vi "Write Test Stand.vi"(8 "error in (no error)":errorcluster, 10 "Generic Test Stand.lvclass":refnum<class "Generic Test Stand.lvclass">, 11 "Run DAC Front Panel in":refnum<class "Run DAC Front Panel.lvclass">) -> (0 "error out":errorcluster, 3 "Run DAC Front Panel out":refnum<class "Run DAC Front Panel.lvclass">)   [LabVIEW 2019, in "DAC Process.lvlib" / "Run DAC Front Panel.lvclass"]
uses:
  Run DAC Front Panel.lvclass
  Generic Test Stand/Generic Test Stand.lvclass
  Run DAC Front Panel.lvclass/Run DAC Front Panel.ctl
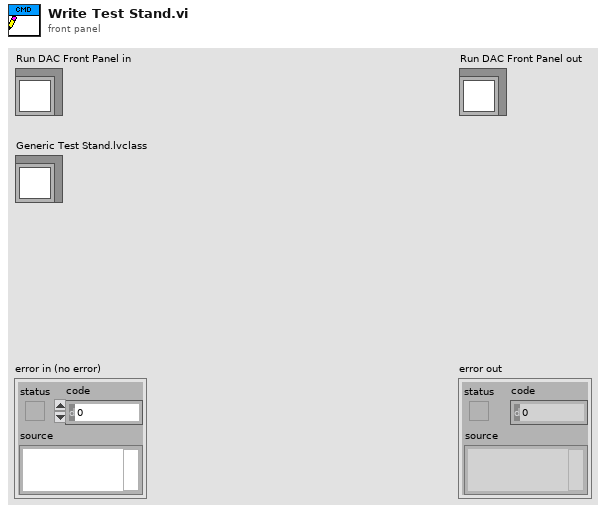
[diagram p1: front panel]
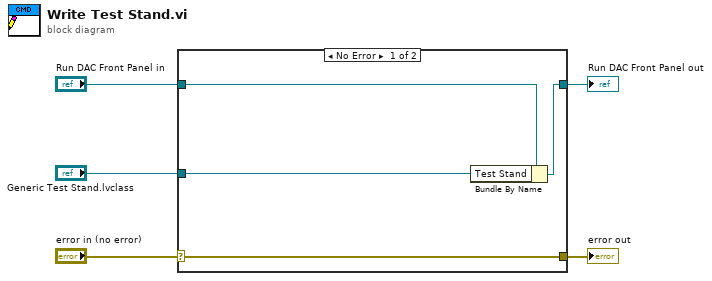
[diagram p0: block diagram]
diagram:
  n1 = case shown="No Error" "error in (no error)" {
    selector: "error in (no error)" -> [w9 w10]
    tunnel: [w9 w10] -> w4
    tunnel: [w7 w11] -> w2
    tunnel: "Run DAC Front Panel in" -> [w8 w11]
    tunnel: "Generic Test Stand.lvclass" -> [w6 _]
    frame No Error {
      n2 = Bundle By Name(cluster=w8, "Test Stand"=w6) -> (w7:refnum<class "Run DAC Front Panel.lvclass">)
    }
    frame Error {
    }
  }
  "error out" <- w4
  "Run DAC Front Panel out" <- w2
